vi "16 TX tester.vi"() -> ()   [LabVIEW 2022 SP3]
panel:
  out "tx free":bool[](array[boolean])=[TRUE, TRUE, TRUE, TRUE, FALSE, FALSE, FALSE, FALSE, FALSE, FALSE, FALSE, FALSE, FALSE, FALSE, FALSE, FALSE]
  out "pulse transmitted":u32=1
  out "fpga clock":u64=191
  in  "file path":path=path "C:/Users/NI/Documents/chaim/chaim_rx/chaim_data/IQ.tdms"
  in  "tdms pulse istraction file path":path=path "C:/Users/NI/Documents/chaim/chaim_rx/chaim_data/pulses.tdms"
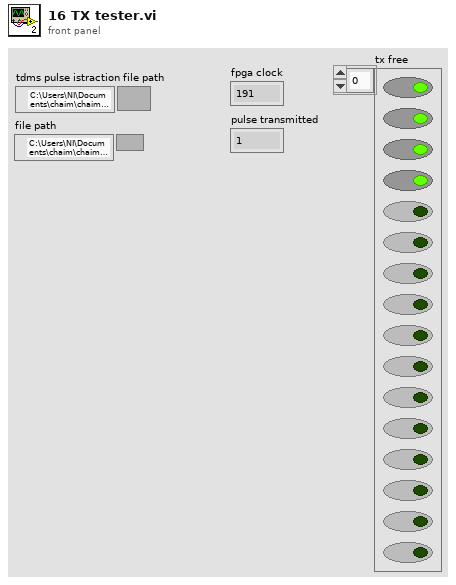
[diagram p1: front panel]
types:
  T1 = enum16{"open", "open or create", "create or replace", "create", "open (read-only)"}
  T2 = typedef "niInstr DSP v1 Shared.lvlib/IQ Data.ctl" = cluster{"I":fxp<+/-,18,1>, "Q":fxp<+/-,18,1>, "overflow":bool}
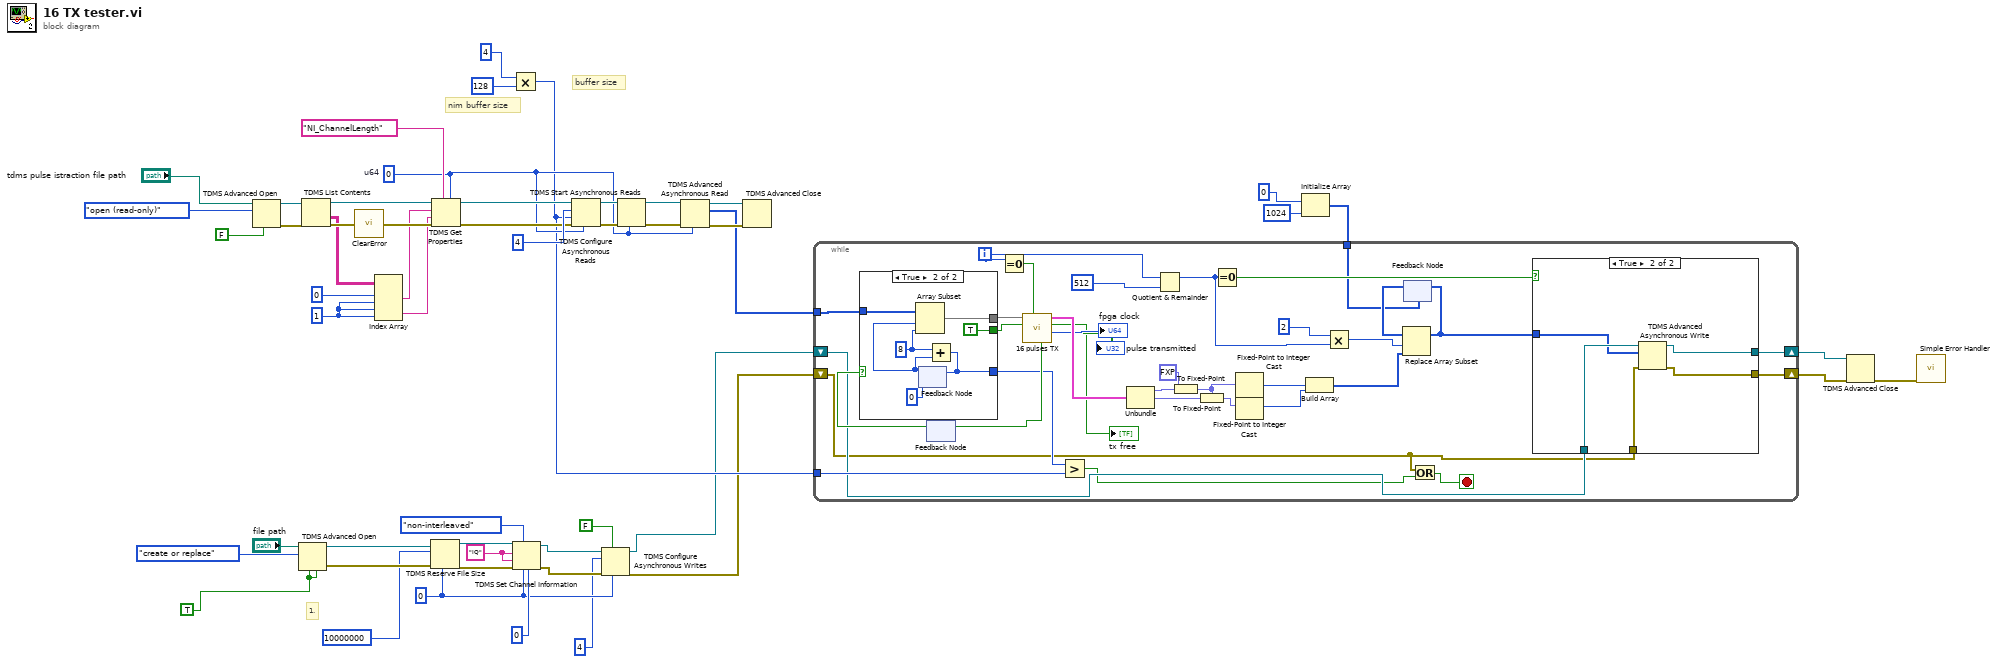
[diagram p0: block diagram]
diagram:
  w8 = TRUE ("disable buffering? (T)")
  w19 = "IQ" ("group name (Untitled)")
  w3 = i16 0 ("data type")
  w39 = 1 ("disabled index (col)")
  w31 = u64 0  # u64
  # "1."
  # "buffer size"
  # "nim buffer size"
  n1 = TDMS Advanced Open(6:FALSE ("Disable Buffering? (T)"), 10:T1."open (read-only)" ("Operation"), 11:"tdms pulse istraction file path") -> (0:w47:errorcluster, 3:w42:refnum<k34>)  [unwired: 2 in, 1 out]
  n2 = TDMS Advanced Open(4:w8, 6:w8, 10:T1."create or replace" ("operation (0:open)"), 11:"file path") -> (0:w22:errorcluster, 3:w23:refnum<k34>)  [unwired: 1 in, 1 out]
  n3 = TDMS List Contents(4:w47, 7:w42) -> (0:w45:errorcluster, 1:w38:string[][], 3:w43:refnum<k34>)  [unwired: 1 in, 1 out]
  n4 = call <vilib>:"ClearError.vi"("error in (no error)"=w45) -> ("error out"=w48:errorcluster)
  n5 = Index Array(array=w38, index (row) #1=0 ("index (row)"), index (col) #1=w39, index (row) #2=w39, index (col) #2=w39) -> (element #1=w37:string, element #2=w36:string)
  n6 = TDMS Reserve File Size(6:w3, 8:w22, 10:u64 10000000 ("reserve size"), 11:w23) -> (0:w20:errorcluster, 3:w21:refnum<k34>)  [unwired: 1 in]
  n7 = TDMS Get Properties(5:w31, 7:"NI_ChannelLength" ("property name"), 8:w48, 9:w36, 10:w37, 11:w43) -> (0:w46:errorcluster, 3:w41:refnum<k34>)  [unwired: 4 out]
  n8 = Multiply(x=u32 4, y=u32 128 ("buffer size")) -> (x*y=w25:u32)
  n9 = TDMS Set Channel Information(4:u32 0 ("samples per channel"), 6:w3, 7:enum16{"non-interleaved", "interleaved"}."non-interleaved" ("data layout (0:non-interleaved)"), 8:w20, 9:w19, 10:w19, 11:w21) -> (0:w4:errorcluster, 3:w7:refnum<k34>)
  n10 = TDMS Configure Asynchronous Reads(6:w31, 8:w46, 9:w25, 10:u32 4 ("Number of Buffers (4)"), 11:w41) -> (0:w50:errorcluster, 3:w35:refnum<k34>)  [unwired: 1 in]
  n11 = TDMS Configure Asynchronous Writes(6:w3, 7:FALSE ("pre-allocate? (F)"), 8:w4, 10:u32 4 ("max asynchronous writes (4)"), 11:w7) -> (0:w5:errorcluster, 3:w6:refnum<k34>)  [unwired: 2 in]
  n12 = TDMS Start Asynchronous Reads(6:w31, 8:w50, 11:w35) -> (0:w30:errorcluster, 3:w29:refnum<k34>)  [unwired: 1 in]
  n13 = TDMS Advanced Asynchronous Read(6:w31, 8:w30, 11:w29) -> (0:w27:errorcluster, 2:w26:u64[], 3:w28:refnum<k34>)  [unwired: 1 out]
  n14 = TDMS Advanced Close(8:w27, 11:w28) -> ()  [unwired: 2 in, 2 out]
  n15 = Initialize Array(i16 0, 1024 ("dimension size")) -> (w9:i16[])
  n16 = while {
    tunnel: w26 -> [w85]
    tunnel: w25 -> [w81]
    shift-right: [w63] -> w16
    shift-left: w5 -> [w55]
    shift-right: [w64] -> w17
    shift-left: w6 -> [w59]
    tunnel: w9 -> [w56]
    i -> [w58]
    stop <- w53 stop-if-true
    n17 = feedback #1() -> (w86:bool)  [unwired: 1 in]
    n18 = case shown="True" w86 {
      tunnel: w85 -> [_ w101]
      tunnel: [_ w98] -> w84
      tunnel: [_ TRUE ("input Valid")] -> w83
      tunnel: [_ w96] -> w82
      frame False {
      }
      frame True {
        w100 = 8 ("length")
        n19 = feedback #2(0) -> (w95:i32)
        n20 = Array Subset(array=w101, index=w95, length=w100) -> (w98:u64[])
        n21 = Add(x=w100, y=w95) -> (x+y=w96:i32)
        n22 = feedback-in #2(w96) -> ()
      }
    }
    n23 = Equal To 0?(x=w58) -> (x = 0?=w57:bool)
    n24 = call "16 pulses TX.vi"("reset system clock"=w57, "PDW input Valid"=w83, "array PDW"=w84) -> ("dds free"=→"pulse transmitted":bool[], "fpga clock"=→"fpga clock":u64, "output valid"=→"tx free":bool, "RF OUT"=w77:T2, "ready for input"=w87:bool)  [unwired: 3 in, 1 out]
    n25 = feedback-in #1(w87) -> ()
    n26 = Greater?(x=w82, y=w81) -> (0:w54:bool)
    n27 = Unbundle(w77) -> ("I"=w78:fxp<+/-,18,1>, "Q"=w76:fxp<+/-,18,1>)  [unwired: 1 out]
    n28 = Quotient & Remainder(x=w58, y=512) -> (x-y*floor(x/y)=w69:i32)  [unwired: 1 out]
    n29 = To Fixed-Point(fixed-point type=fxp<+/-,16,1> 0.0, number=w78) -> (fixed-point=w74:fxp<+/-,16,1>)
    n30 = To Fixed-Point(fixed-point type=w74, number=w76) -> (fixed-point=w73:fxp<+/-,16,1>)
    n31 = Equal To 0?(x=w69) -> (x = 0?=w66:bool)
    n32 = Fixed-Point to Integer Cast(1:w74) -> (0:w72:i16)
    n33 = Fixed-Point to Integer Cast(1:w73) -> (0:w71:i16)
    n34 = Build Array(w72, w71) -> (w70:i16[])
    n35 = Multiply(x=2, y=w69) -> (x*y=w67:i32)
    n36 = feedback #3(w56) -> (w79:i16[])
    n37 = Replace Array Subset(array=w79, new element=w70, index=w67) -> (w65:i16[])
    n38 = feedback-in #3(w65) -> ()
    n39 = Or(x=w55, y=w54) -> (x .or. y?=w53:bool)
    n40 = case shown="True" w66 {
      tunnel: w59 -> [w89 w94]
      tunnel: w55 -> [w88 w93]
      tunnel: w65 -> [_ w92]
      tunnel: [w89 w91] -> w64
      tunnel: [w88 w90] -> w63
      frame False {
      }
      frame True {
        n41 = TDMS Advanced Asynchronous Write(8:w93, 10:w92, 11:w94) -> (0:w90:errorcluster, 3:w91:refnum<k34>)
      }
    }
  }
  n42 = TDMS Advanced Close(8:w16, 11:w17) -> (0:w18:errorcluster)  [unwired: 2 in, 1 out]
  n43 = call <vilib>:"Simple Error Handler.vi"("error in (no error)"=w18) -> ()  [unwired: 1 in, 8 out]
